vi "test_sync-coords.vi"() -> ()   [LabVIEW 2010]
panel:
  out "Connected":bool
  out "Open Automation Error":errorcluster
  out "NO":bool
  out "DEC TMP":dbl format="%.6g"
  out "RA TMP":dbl format="%.6g"
  in  "DEC TEL":dbl format="%.6g"
  in  "RA TEL":dbl format="%.6g"
  out "DEC SN":dbl format="%.6g"
  out "RA SN":dbl format="%.6g"
  in  "Quit":bool
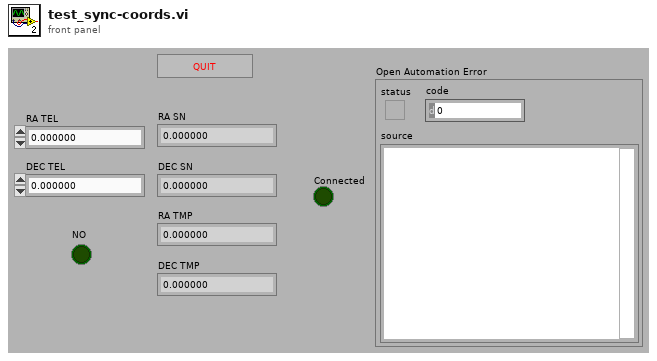
[diagram p1: front panel]
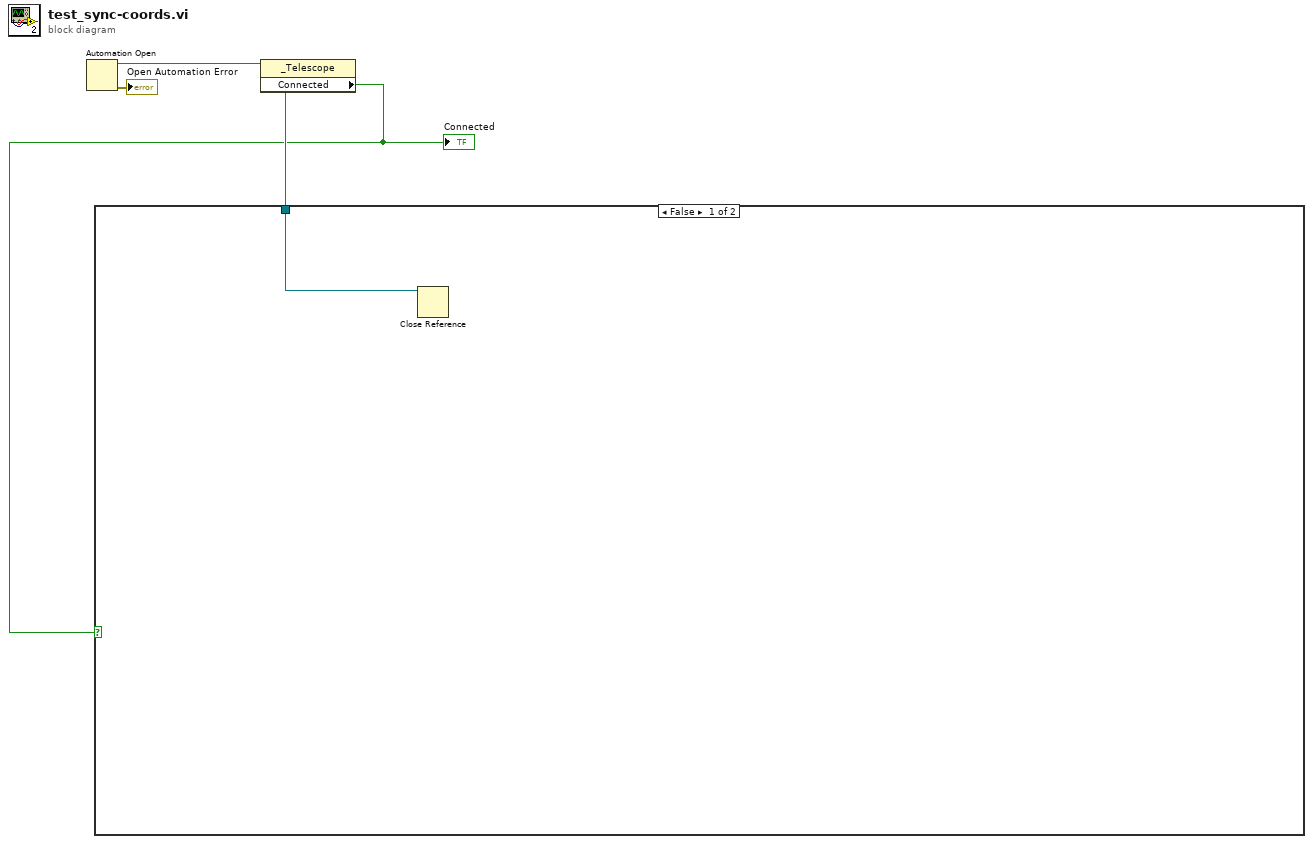
[diagram p0: block diagram]
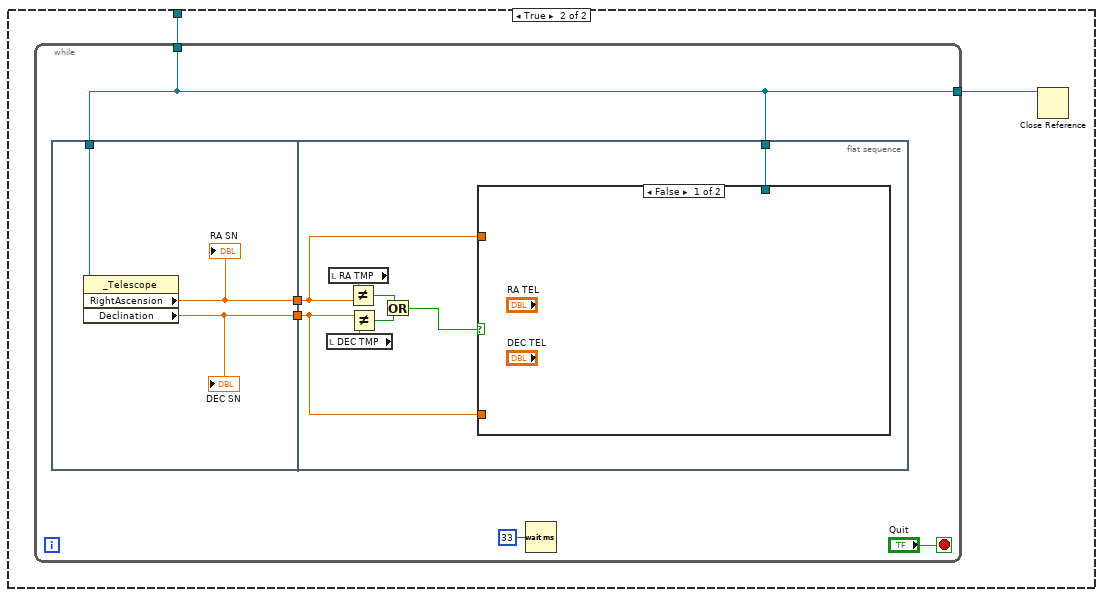
[diagram p2: hidden frame]
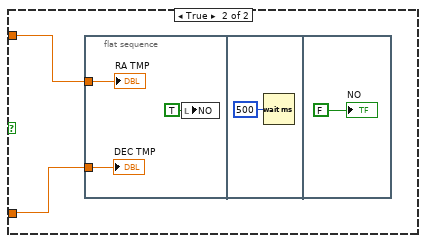
[diagram p3: hidden frame]
diagram:
  n1 = Automation Open() -> (Automation Refnum=w2:refnum<k7>, error out=→"Open Automation Error":errorcluster)  [unwired: 4 in]
  n2 = property class="_Telescope"(reference=w2) -> ("Connected"=w1:bool)  [unwired: 1 in, 2 out]
  "Connected" <- w1
  n3 = case shown="False" w1 {
    tunnel: w2 -> [w4 w6]
    frame False {
      n4 = Close Reference(reference=w4) -> ()  [unwired: 1 in, 1 out]
    }
    frame True {
      n5 = while {
        tunnel: w6 -> [w7]
        tunnel: [w7] -> w5
        stop <- "Quit" stop-if-true
        n6 = flat-sequence {
          tunnel: w7 -> [w14]
          tunnel: [w13] -> w9
          tunnel: [w12] -> w8
          tunnel: w7 -> [w22]
          tunnel: w9 -> [w15]
          tunnel: w8 -> [w16]
          frame #0 {
            n7 = property class="_Telescope"(reference=w14) -> ("RightAscension"=w13:dbl, "Declination"=w12:dbl)  [unwired: 1 in, 2 out]
            "RA SN" <- w13
            "DEC SN" <- w12
          }
          frame #1 {
            n8 = local read "DEC TMP"() -> (w20:dbl)
            n9 = local read "RA TMP"() -> (w21:dbl)
            n10 = Not Equal?(x=w21, y=w15) -> (x != y?=w19:bool)
            n11 = Not Equal?(x=w16, y=w20) -> (x != y?=w18:bool)
            n12 = Or(x=w19, y=w18) -> (x .or. y?=w17:bool)
            n13 = case shown="False" w17 {
              tunnel: w22 -> [_ _]
              tunnel: w16 -> [_ w23]
              tunnel: w15 -> [_ w24]
              frame False {
              }
              frame True {
                n14 = flat-sequence {
                  tunnel: w24 -> [w26]
                  tunnel: w23 -> [w25]
                  frame #0 {
                    n15 = local write "NO"(TRUE) -> ()
                    "DEC TMP" <- w25
                    "RA TMP" <- w26
                  }
                  frame #1 {
                    n16 = Wait (ms)(milliseconds to wait=u32 500) -> ()  [unwired: 1 out]
                  }
                  frame #2 {
                    "NO" <- FALSE
                  }
                }
              }
            }
          }
        }
        n17 = Wait (ms)(milliseconds to wait=u32 33) -> ()  [unwired: 1 out]
      }
      n18 = Close Reference(reference=w5) -> ()  [unwired: 1 in, 1 out]
    }
  }
